vi "memory_load_B_1.vi"() -> (0 "Init Data Out":fxp<+/-,32,16>[](array[numeric]))   [LabVIEW 2020]
panel:
  out "size(s)":i32
  # "For Initialization VI requirements and help, please read directions located on Block Diagram."
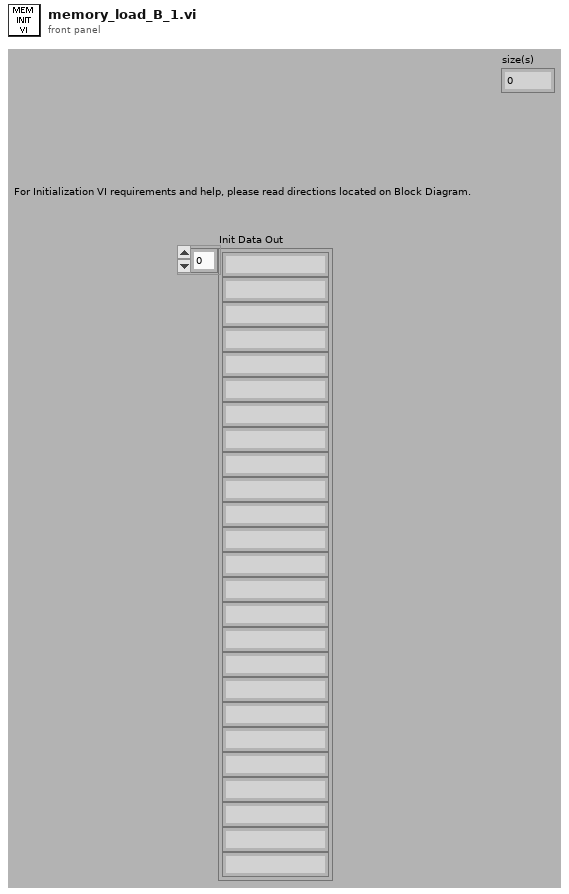
[diagram p1: front panel]
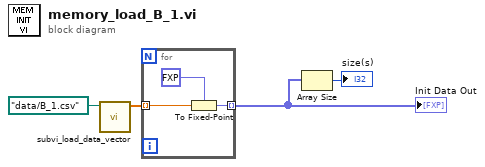
[diagram p0: block diagram]
diagram:
  n1 = call "subvi_load_data_vector.vi"("default name"=path "data/B_1.csv") -> ("array type (2D Dbl) out"=w3:dbl[])  [unwired: 10 in]
  n2 = for {
    tunnel: w3 -> [w7] mode=indexing
    tunnel: [w6] -> w2 mode=indexing
    n3 = To Fixed-Point(fixed-point type=fxp<+/-,32,16> 0.0 ("fixed-point"), number=w7) -> (fixed-point=w6:fxp<+/-,32,16>)
  }
  "Init Data Out" <- w2
  n4 = Array Size(array=w2) -> (size(s)=→"size(s)":i32)
